vi "DT_Triangle Manager_Format Ghost.vi"(6 "triangle":i32, 8 "p 2 triangle":i32, 9 "p 1 triangle":i32, 10 "p 2":i32, 11 "p 1":i32) -> (3 "Triangle":i32[](array[numeric]))   [LabVIEW 2017, in "NI_AAL_Geometry.lvlib"]
uses:
  <vilib>/Analysis/NI_AAL_Geometry.lvlib
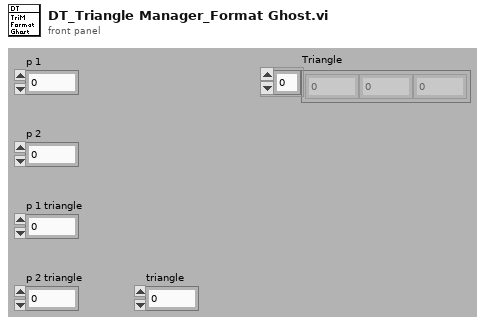
[diagram p1: front panel]
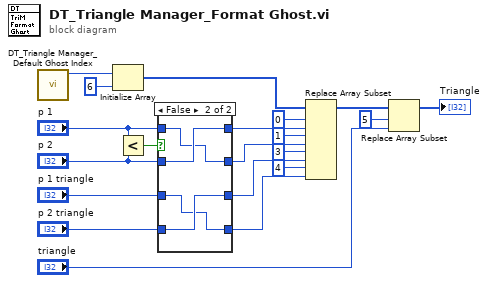
[diagram p0: block diagram]
diagram:
  n1 = call <vilib>:"DT_Triangle Manager_Default Ghost Index.vi"() -> ("ghost index"=w19:i32)  [unwired: 11 out]
  n2 = Initialize Array(w19, 6 ("dimension size")) -> (w5:i32[])
  n3 = Less?(x="p 1", y="p 2") -> (x < y?=w20:bool)
  n4 = case shown="False" w20 {
    tunnel: "p 1" -> [w21 w25]
    tunnel: "p 2" -> [w22 w26]
    tunnel: "p 1 triangle" -> [w24 w27]
    tunnel: "p 2 triangle" -> [w23 w28]
    tunnel: [w24 w28] -> w4
    tunnel: [w23 w27] -> w3
    tunnel: [w22 w25] -> w2
    tunnel: [w21 w26] -> w1
    frame True {
    }
    frame False {
    }
  }
  n5 = Replace Array Subset(array=w5, new element #1=w1, index #1=0 ("index"), new element #2=w2, index #2=1 ("index"), new element #3=w4, index #3=3 ("index"), new element #4=w3, index #4=4 ("index")) -> (w6:i32[])
  n6 = Replace Array Subset(array=w6, new element="triangle", index=5) -> (→"Triangle":i32[])
